vi "Control Reference To Array Of Variants.vi"(4 "Registry Variant Accessor":refnum<class "CConfig Variant Accessor.lvclass">, 6 "Controls":refnum<vi>[](array[refnum]), 8 "error in (no error)":errorcluster, 11 "Registry Control Reference Accessor in":refnum<class "Registry Ctrl Ref Accessor.lvclass">) -> (0 "error out":errorcluster, 1 "Variants":variant[](array[variant]), 2 "Controls":refnum<vi>[](array[refnum]), 3 "Registry Control Reference Accessor out":refnum<class "Registry Ctrl Ref Accessor.lvclass">)   [LabVIEW 2013, in "Registry Ctrl Ref Accessor.lvclass"]
doc: "Copyright 2018, Carya Automatisering, Wiebe Walstra."
uses:
  Registry Ctrl Ref Accessor.lvclass
  CConfig Variant Accessor/CConfig Variant Accessor.lvclass
  Registry Ctrl Ref Accessor.lvclass/Registry Ctrl Ref Accessor.ctl
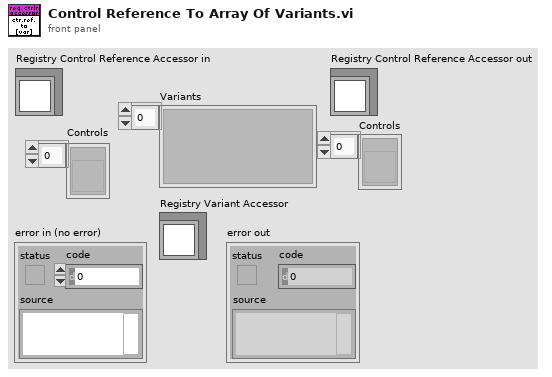
[diagram p1: front panel]
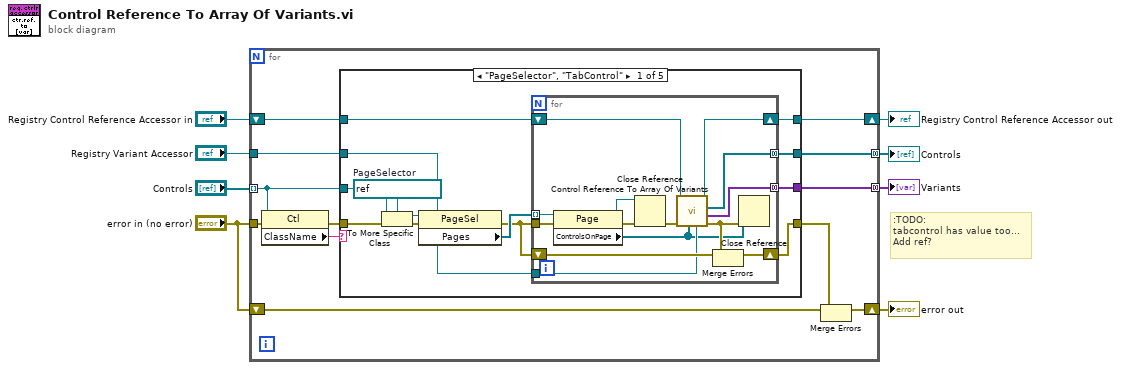
[diagram p0: block diagram]
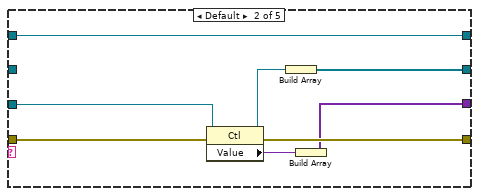
[diagram p2: hidden frame]
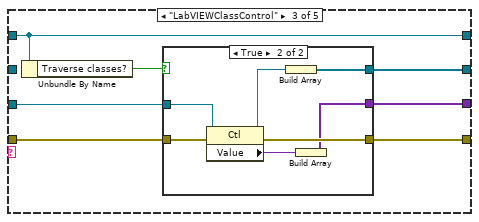
[diagram p3: hidden frame]
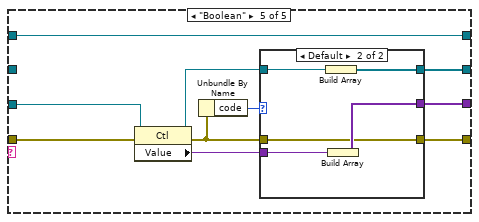
[diagram p6: hidden frame]
diagram:
  # ":TODO:\ntabcontrol has value too...\nAdd ref?"
  n1 = for {
    tunnel: "error in (no error)" -> [w20]
    tunnel: "Controls" -> [w18] mode=indexing
    shift-right: [w15] -> w6
    shift-left: "error in (no error)" -> [w17]
    shift-right: [w14] -> w5
    shift-left: "Registry Control Reference Accessor in" -> [w13]
    tunnel: [w11] -> w2 mode=concatenating
    tunnel: "Registry Variant Accessor" -> [w12]
    tunnel: [w10] -> w1 mode=concatenating
    n2 = property class="Ctl"(reference=w18, error in=w20) -> (error out=w19:errorcluster, "ClassName"=w9:string)  [unwired: 1 out]
    n3 = case shown="\"PageSelector\", \"TabControl\"" w9 {
      tunnel: [w26 w55 w62 w71 w73] -> w16
      tunnel: w19 -> [w33 w50 w58 w71 w79]
      tunnel: w18 -> [w31 w53 w61 _ w76]
      tunnel: w13 -> [w25 w54 w57 w72 w82]
      tunnel: [w24 w54 w57 w72 w82] -> w14
      tunnel: w12 -> [w23 _ _ _ _]
      tunnel: [w22 w52 w60 _ w81] -> w11
      tunnel: [w21 w51 w59 _ w80] -> w10
      frame "PageSelector", "TabControl" {
        w29 = refnum<vi> refnum  # PageSelector
        n4 = To More Specific Class(target class=w29, reference=w31, error in=w33) -> (specific class reference=w30:refnum<vi>, error out=w32:errorcluster)
        n5 = property class="PageSel"(reference=w30, error in=w32) -> (error out=w27:errorcluster, "Pages"=w28:refnum<vi>[])  [unwired: 1 out]
        n6 = for {
          tunnel: w28 -> [w47] mode=indexing
          tunnel: w27 -> [w46]
          shift-right: [w44] -> w26
          shift-left: w27 -> [w45]
          shift-right: [w38] -> w24
          shift-left: w25 -> [w39]
          tunnel: [w36] -> w22 mode=concatenating
          tunnel: w23 -> [w37]
          tunnel: [w34] -> w21 mode=concatenating
          n7 = property class="Page"(reference=w47, error in=w46) -> (reference out=w40:refnum<vi>, error out=w42:errorcluster, "ControlsOnPage"=w35:refnum<vi>[])
          n8 = Close Reference(reference=w40, error in (no error)=w42) -> (error out=w41:errorcluster)
          n9 = call-dynamic "Control Reference To Array Of Variants.vi"("Registry Variant Accessor"=w37, "Controls"=w35, "error in (no error)"=w41, "Registry Control Reference Accessor in"=w39) -> ("error out"=w43:errorcluster, "Variants"=w36:variant[], "Controls"=w34:refnum<vi>[], "Registry Control Reference Accessor out"=w38:refnum<class "Registry Ctrl Ref Accessor.lvclass">)  [unwired: 4 in]
          n10 = Merge Errors(w45, w43) -> (w44:errorcluster)
          n11 = Close Reference(reference=w35, error in (no error)=w43) -> ()  [unwired: 1 out]
        }
      }
      frame Default {
        n12 = property class="Ctl"(reference=w53, error in=w50) -> (reference out=w48:refnum<vi>, error out=w55:errorcluster, "Value"=w49:variant)
        n13 = Build Array(w48) -> (w51:refnum<vi>[])
        n14 = Build Array(w49) -> (w52:variant[])
      }
      frame "LabVIEWClassControl" {
        n15 = Unbundle By Name(w57) -> ("Traverse classes?"=w56:bool)
        n16 = case shown="True" w56 {
          tunnel: [w63 w70] -> w62
          tunnel: w61 -> [_ w69]
          tunnel: [_ w68] -> w60
          tunnel: [_ w67] -> w59
          tunnel: w58 -> [w63 w66]
          frame False {
          }
          frame True {
            n17 = property class="Ctl"(reference=w69, error in=w66) -> (reference out=w64:refnum<vi>, error out=w70:errorcluster, "Value"=w65:variant)
            n18 = Build Array(w64) -> (w67:refnum<vi>[])
            n19 = Build Array(w65) -> (w68:variant[])
          }
        }
      }
      frame "SubPanel" {
      }
      frame "Boolean" {
        n20 = property class="Ctl"(reference=w76, error in=w79) -> (reference out=w77:refnum<vi>, error out=w74:errorcluster, "Value"=w78:variant)
        n21 = Unbundle By Name(w74) -> ("code"=w75:i32)
        n22 = case shown="Default" w75 {
          tunnel: [_ w87] -> w81
          tunnel: [_ w86] -> w80
          tunnel: w78 -> [_ w85]
          tunnel: w77 -> [_ w84]
          tunnel: w74 -> [_ w83]
          tunnel: [_ w83] -> w73
          frame 1193 {
          }
          frame Default {
            n23 = Build Array(w84) -> (w86:refnum<vi>[])
            n24 = Build Array(w85) -> (w87:variant[])
          }
        }
      }
    }
    n25 = Merge Errors(w17, w16) -> (w15:errorcluster)
  }
  "error out" <- w6
  "Registry Control Reference Accessor out" <- w5
  "Variants" <- w2
  "Controls" <- w1
